vi "INITIALIZE.vi"(8 "error in (no error)":errorcluster, 11 "UI_CAFÉ_MEX_ESP in":refnum<class "UI_CAFÉ_MEX_ESP.lvclass">) -> (0 "error out":errorcluster, 3 "UI_CAFÉ_MEX_ESP out":refnum<class "UI_CAFÉ_MEX_ESP.lvclass">)   [LabVIEW 2019, in "DATA_UI_CAFÉ_MEX_ESP.lvlib" / "UI_CAFÉ_MEX_ESP.lvclass"]
uses:
  Read PRODUCTOS.vi
  Read VI Refnum.vi
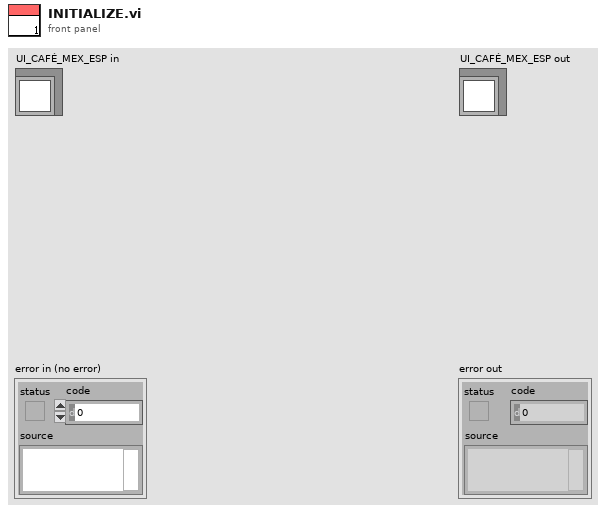
[diagram p1: front panel]
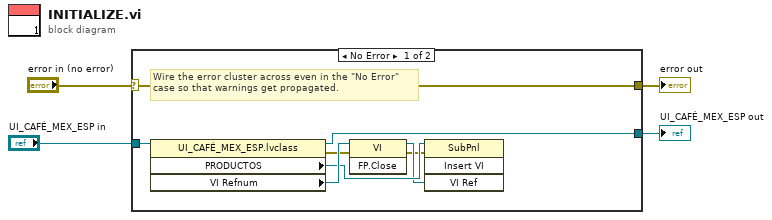
[diagram p0: block diagram]
diagram:
  n1 = case shown="No Error" "error in (no error)" {
    selector: "error in (no error)" -> [w11 w14]
    tunnel: [w11 w14] -> w3
    tunnel: [w10 w13] -> w1
    tunnel: "UI_CAFÉ_MEX_ESP in" -> [w12 w13]
    frame No Error {
      # "Wire the error cluster across even in the \"No Error\"\ncase so that warnings get propagated."
      n2 = property class="UI_CAFÉ_MEX_ESP.lvclass"(reference=w12) -> (reference out=w10:refnum<class "UI_CAFÉ_MEX_ESP.lvclass">, error out=w6:errorcluster, "PRODUCTOS"=w8:refnum<vi>, "VI Refnum"=w9:refnum<vi>)  [unwired: 1 in]
      n3 = invoke class="VI" method="FP.Close"(reference=w9, error in=w6) -> (reference out=w7:refnum<vi>, error out=w5:errorcluster)  [unwired: 1 in, 1 out]
      n4 = invoke class="SubPnl" method="Insert VI"(reference=w8, error in=w5, "VI Ref"=w7) -> ()  [unwired: 1 in, 4 out]
    }
    frame Error {
    }
  }
  "error out" <- w3
  "UI_CAFÉ_MEX_ESP out" <- w1
